vi "initBaslerCamera.vi"(4 "buffer size":i32=5, 5 "camera controls":T4={"Camera Name"="cam0", "exposure time (us)"=10000, "GainRaw"=100, "Red balance"=100, "Green balance"=100, "Blue balance"=100}, 6 "im proc controls":T1={"Color Plane"=2, "downsampling"=24, "Filter"=enum."AutoM", "Number of Erosions"=2, "Focus threshold"=20.0, "Focus std threshold"=0.0, "background\nsubtraction"=FALSE, "Threshold"=0} {"Threshold" scale=0.0..255.0; "Color Plane" items=["Red", "Green", "Blue", "Hue", "Saturation", "Luminance", "Value", "Intensity"]}, 7 "image format controls":T2={"Pixel Format"="YUV 422 Packed", "width"=2500, "height"=900, "sub image height"=2500, "sub image width"=2500}) -> ()   [LabVIEW 2012]
uses:
  <vilib>/userdefined/High Color/IMAQdx.ctl
  GlobalBaslerCamera.vi
  <vilib>/vision/driver/NI_Vision_Acquisition_Software.lvlib
  <resource>/objmgr/imaqdx.rc
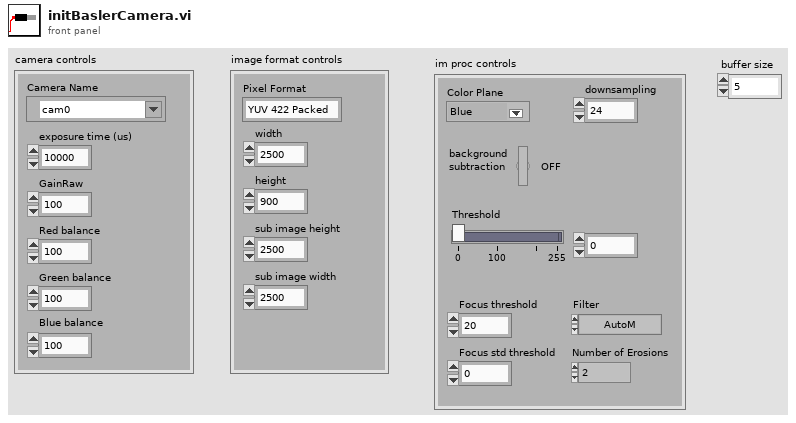
[diagram p1: front panel]
types:
  T1 = cluster{"Color Plane":i32, "downsampling":i32, "Filter":enum32{"AutoM", "Close", "Dilate", "Erode", "Gradient", "Gradient out", "Gradient in", "Hit miss", "Open", "PClose", "POpen", "Thick", "Thin"}, "Number of Erosions":i32, "Focus threshold":sgl, "Focus std threshold":sgl, "background\nsubtraction":bool, "Threshold":u8}
  T2 = cluster{"Pixel Format":string, "width":u32, "height":u32, "sub image height":u32, "sub image width":u32}
  T3 = typedef "IMAQdx.ctl" = refnum<k21>
  T4 = cluster{"Camera Name":T3, "exposure time (us)":u32, "GainRaw":i64, "Red balance":u8, "Green balance":u8, "Blue balance":u8}
  T5 = typedef "Image Type" = u32
  T6 = typedef "IMAQ Image.ctl" = refnum<image>
  T7 = typedef "Semaphore RefNum" = refnum<k1>
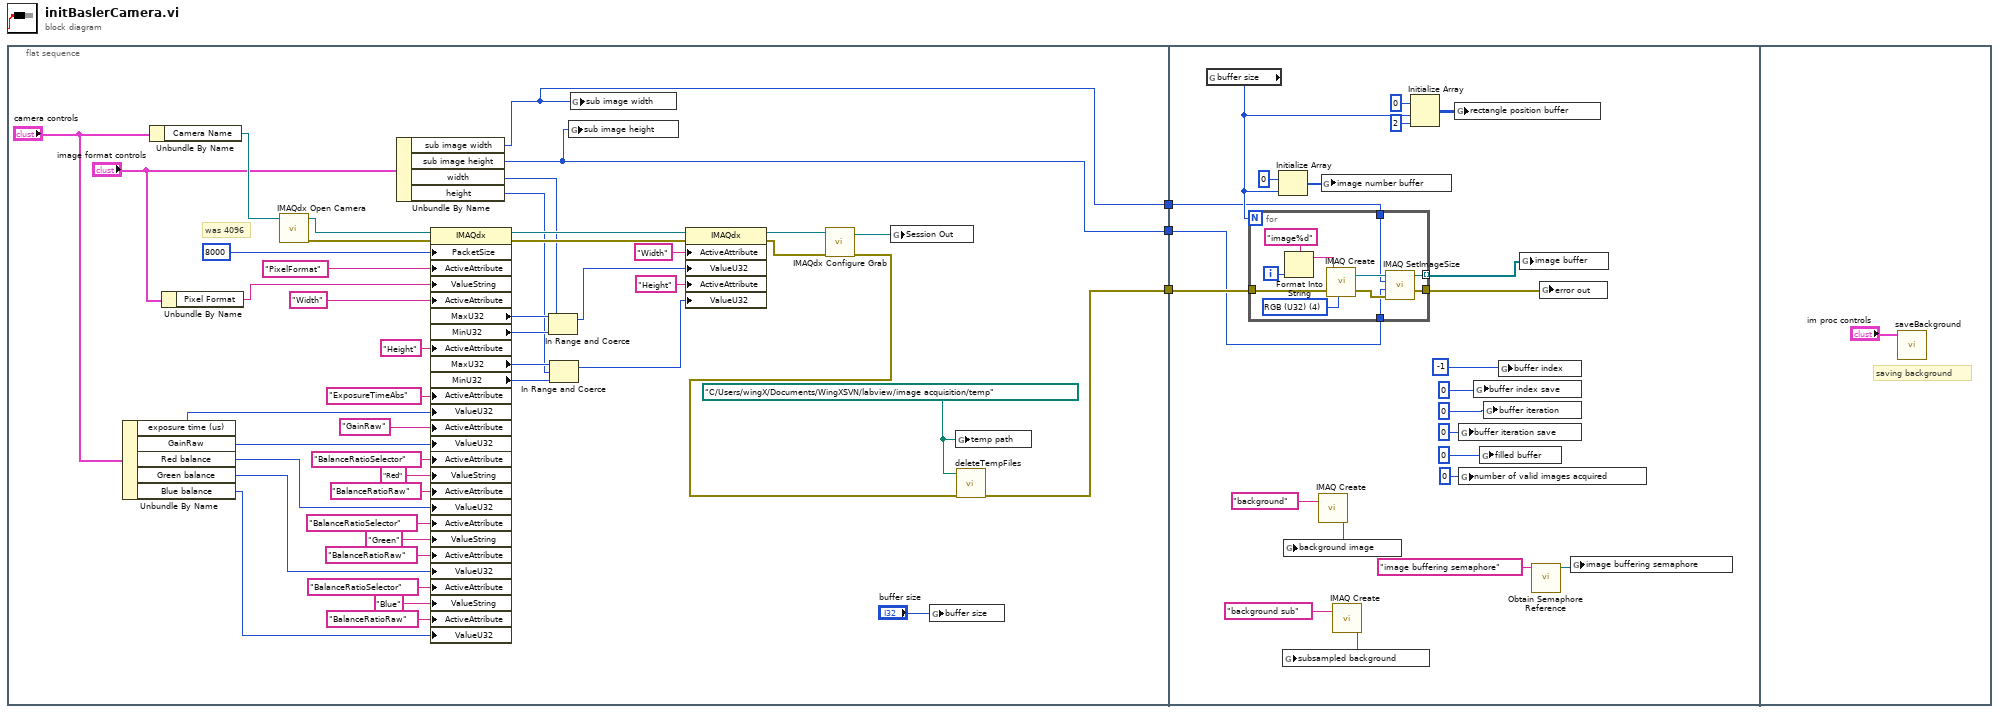
[diagram p0: block diagram]
diagram:
  n1 = flat-sequence {
    tunnel: [w7] -> w3
    tunnel: [w6] -> w2
    tunnel: [w5] -> w1
    tunnel: w3 -> [w68]
    tunnel: w2 -> [w54]
    tunnel: w1 -> [w53]
    frame #0 {
      w34 = path "C:/Users/wingX/Documents/WingXSVN/labview/image acquisition/temp" ("temp path")
      # "was 4096"
      n2 = Unbundle By Name("camera controls") -> ("exposure time (us)"=w26:u32, "GainRaw"=w25:i64, "Red balance"=w21:u8, "Green balance"=w17:u8, "Blue balance"=w13:u8)
      n3 = Unbundle By Name("camera controls") -> ("Camera Name"=w29:T3)
      n4 = Unbundle By Name("image format controls") -> ("Pixel Format"=w32:string)
      n5 = call <vilib>:"IMAQdx Open Camera.vi"("Session In"=w29) -> ("error out"=w49:errorcluster, "Session Out"=w50:T3)  [unwired: 2 in, 7 out]
      n6 = Unbundle By Name("image format controls") -> ("sub image width"=w6:u32, "sub image height"=w5:u32, "width"=w31:u32, "height"=w30:u32)
      n7 = property class="IMAQdx"(reference=w50, error in=w49, "PacketSize"=u32 8000, "ActiveAttribute"="PixelFormat", "ValueString"=w32, "ActiveAttribute"="Width", "ActiveAttribute"="Height", "ActiveAttribute"="ExposureTimeAbs", "ValueU32"=w26, "ActiveAttribute"="GainRaw", "ValueU32"=w25, "ActiveAttribute"="BalanceRatioSelector", "ValueString"="Red", "ActiveAttribute"="BalanceRatioRaw", "ValueU32"=w21, "ActiveAttribute"="BalanceRatioSelector", "ValueString"="Green", "ActiveAttribute"="BalanceRatioRaw", "ValueU32"=w17, "ActiveAttribute"="BalanceRatioSelector", "ValueString"="Blue", "ActiveAttribute"="BalanceRatioRaw", "ValueU32"=w13) -> (reference out=w40:T3, error out=w39:errorcluster, "MaxU32"=w45:u32, "MinU32"=w44:u32, "MaxU32"=w42:u32, "MinU32"=w41:u32)
      n8 = In Range and Coerce(upper limit=w45, x=w31, lower limit=w44) -> (coerced(x)=w10:u32)  [unwired: 1 out]
      n9 = In Range and Coerce(upper limit=w42, x=w30, lower limit=w41) -> (coerced(x)=w8:u32)  [unwired: 1 out]
      n10 = global write "GlobalBaslerCamera.vi" "sub image height"(w5) -> ()
      n11 = global write "GlobalBaslerCamera.vi" "sub image width"(w6) -> ()
      n12 = property class="IMAQdx"(reference=w40, error in=w39, "ActiveAttribute"="Width", "ValueU32"=w10, "ActiveAttribute"="Height", "ValueU32"=w8) -> (reference out=w38:T3, error out=w37:errorcluster)
      n13 = call <vilib>:"IMAQdx Configure Grab.vi"("error in"=w37, "Session In"=w38) -> ("error out"=w33:errorcluster, "Session Out"=w35:T3)  [unwired: 8 out]
      n14 = global write "GlobalBaslerCamera.vi" "Session Out"(w35) -> ()
      n15 = global write "GlobalBaslerCamera.vi" "buffer size"("buffer size") -> ()
      n16 = global write "GlobalBaslerCamera.vi" "temp path"(w34) -> ()
      n17 = call "deleteTempFiles.vi"("error in"=w33, "path"=w34) -> ("error out"=w7:errorcluster)  [unwired: 7 in]
    }
    frame #1 {
      n18 = global read "GlobalBaslerCamera.vi" "buffer size"() -> (w64:i32)
      n19 = for {
        N: w64 -> [_]
        tunnel: w68 -> [w84]
        tunnel: [w78] -> w67 mode=indexing
        tunnel: [w76] -> w69
        tunnel: w54 -> [w75]
        tunnel: w53 -> [w74]
        i -> [w83]
        w80 = T5 4 items=["Grayscale (U8)", "Grayscale (I16)", "Grayscale (SGL)", "Complex (CSG)", "RGB (U32)", "HSL (U32)", "RGB (U64)", "Grayscale (U16)"] ("Image Type")
        n20 = Format Into String(format string="image%d" ("Image Name"), w83) -> (resulting string=w82:string)  [unwired: 2 in, 1 out]
        n21 = call "IMAQ Create"("Image Name"=w82, "Image Type"=w80, "error in (no error)"=w84) -> ("New Image"=w79:T6, "error out"=w77:errorcluster)  [unwired: 1 in, 1 out]
        n22 = call "IMAQ SetImageSize"("error in (no error)"=w77, "Y Resolution"=w74, "X Resolution"=w75, "Image"=w79) -> ("error out"=w76:errorcluster, "Image Out"=w78:T6)  [unwired: 1 in]
      }
      n23 = Initialize Array(u16 0 ("element"), w64) -> (w65:u16[])
      n24 = call "IMAQ Create"("Image Name"="background") -> ("New Image"=w72:T6)  [unwired: 3 in, 2 out]
      n25 = global write "GlobalBaslerCamera.vi" "background image"(w72) -> ()
      n26 = global write "GlobalBaslerCamera.vi" "image number buffer"(w65) -> ()
      n27 = call "IMAQ Create"("Image Name"="background sub") -> ("New Image"=w70:T6)  [unwired: 3 in, 2 out]
      n28 = global write "GlobalBaslerCamera.vi" "subsampled background"(w70) -> ()
      n29 = Initialize Array(u16 0 ("element"), w64, 2 ("dimension size")) -> (w61:u16[][])
      n30 = global write "GlobalBaslerCamera.vi" "rectangle position buffer"(w61) -> ()
      n31 = global write "GlobalBaslerCamera.vi" "buffer iteration save"(0 ("buffer index")) -> ()
      n32 = global write "GlobalBaslerCamera.vi" "number of valid images acquired"(0 ("number of valid images acquired")) -> ()
      n33 = global write "GlobalBaslerCamera.vi" "buffer index save"(0 ("buffer index")) -> ()
      n34 = global write "GlobalBaslerCamera.vi" "filled buffer"(0 ("buffer index")) -> ()
      n35 = global write "GlobalBaslerCamera.vi" "buffer iteration"(0 ("buffer index")) -> ()
      n36 = global write "GlobalBaslerCamera.vi" "buffer index"(-1 ("buffer index")) -> ()
      n37 = global write "GlobalBaslerCamera.vi" "image buffer"(w67) -> ()
      n38 = call <vilib>:"Obtain Semaphore Reference.vi"("name (unnamed)"="image buffering semaphore") -> ("semaphore"=w51:T7)  [unwired: 4 in, 2 out]
      n39 = global write "GlobalBaslerCamera.vi" "error out"(w69) -> ()
      n40 = global write "GlobalBaslerCamera.vi" "image buffering semaphore"(w51) -> ()
    }
    frame #2 {
      # "saving background"
      n41 = call "saveBackground.vi"("im proc controls"="im proc controls") -> ()  [unwired: 11 in]
    }
  }
